vi "2-input AND.vi"(10 "Obtained Expression":string, 11 "Input List":string[](array[string])) -> (1 "O/p = I/p":string, 2 "AND ?":bool, 3 "Logic Exp":string)   [LabVIEW 2014]
doc: "This VI is used to compare the obtained logic with the logic of NAND gate."
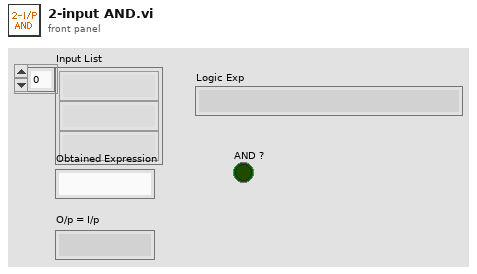
[diagram p1: front panel]
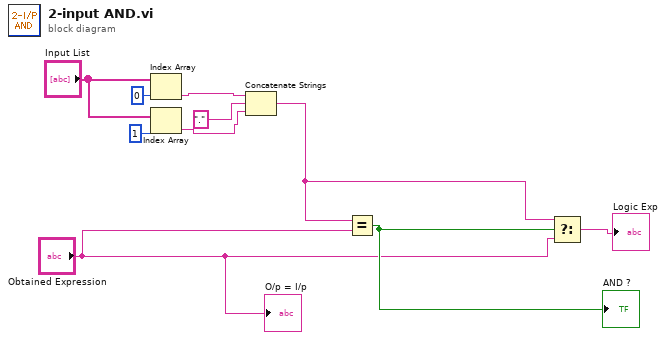
[diagram p0: block diagram]
diagram:
  n1 = Index Array(array="Input List", index=0) -> (element=w8:string)
  n2 = Index Array(array="Input List", index=1) -> (element=w10:string)
  n3 = Concatenate Strings(w8, "." ("string"), w10) -> (w2:string)
  n4 = Equal?(x=w2, y="Obtained Expression") -> (x = y?=w5:bool)
  "AND ?" <- w5
  n5 = Select(t=w2, s=w5, f="Obtained Expression") -> (s? t:f=→"Logic Exp":string)
  "O/p = I/p" <- "Obtained Expression"
